vi "QueueToCommand.vi"(0 "ROS":T1={"topic port"=1236, "Node"="/labview", "topic"="/robot/head/command_head_nod", "type"="std_msgs/Bool", "node port"=7000, "error "={"status"=FALSE, "code"=0, "source"=""}, "Direction"=enum."Publisher", "Update (ms)"=1, "FIFO size"=1}, 2 "Check":enum16{"Cmd+Write", "FIFO", "CMD", "CMD /wait"}(ring)) -> (3 "ROS out":T1={"topic port"=1236, "Node"="/labview", "topic"="/robot/head/command_head_nod", "type"="std_msgs/Bool", "node port"=7000, "error "={"status"=FALSE, "code"=0, "source"=""}, "Direction"=enum."Publisher", "Update (ms)"=1, "FIFO size"=1}, 4 "Command":string, 5 "Queue log":string, 6 "data":string)   [LabVIEW 2014]
doc: "Executes a command from the queue"
uses:
  SubVIs/_ROSControl.ctl
  SubVIs/_ROSDirection.ctl
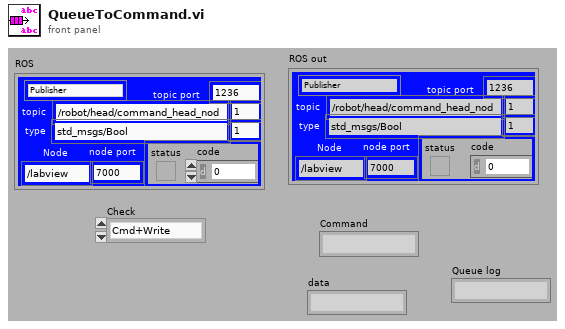
[diagram p1: front panel]
types:
  T1 = typedef "_ROSControl.ctl" = cluster{"topic port":u16, "Node":string, "topic":string, "type":string, "node port":u16, "error ":errorcluster, "Direction":T2, "Update (ms)":u16, "FIFO size":u16}
  T2 = typedef "_ROSDirection.ctl" = enum16{"Node", "Publisher", "Subscriber", "ServiceClient", "ServiceProvider"}
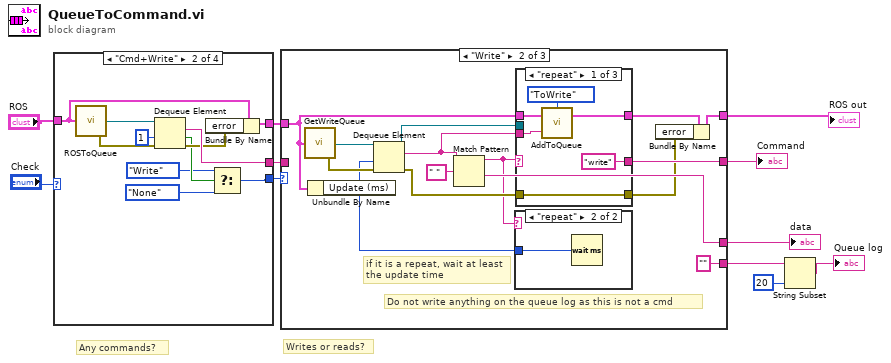
[diagram p0: block diagram]
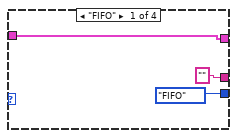
[diagram p2: hidden frame]
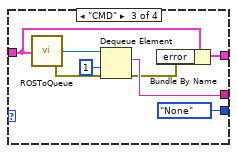
[diagram p3: hidden frame]
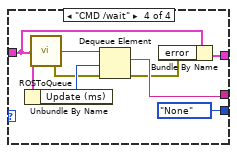
[diagram p4: hidden frame]
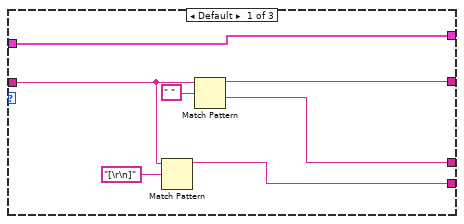
[diagram p5: hidden frame]
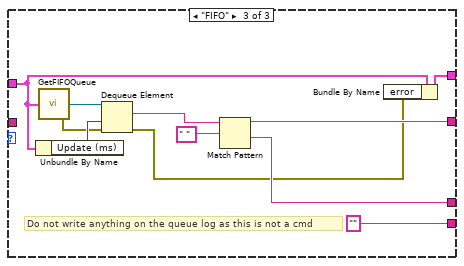
[diagram p9: hidden frame]
diagram:
  # "Writes or reads?"
  # "Any commands?"
  n1 = case shown="\"Cmd+Write\"" "Check" {
    tunnel: [enum16{"FIFO", "Write", "None"}."FIFO" w15 enum16{"FIFO", "Write", "None"}."None" enum16{"FIFO", "Write", "None"}."None"] -> w11
    tunnel: "ROS" -> [w13 w21 w29 w37]
    tunnel: ["" w23 w32 w40] -> w8
    tunnel: [w13 w20 w28 w36] -> w2
    frame "FIFO" {
    }
    frame "Cmd+Write" {
      n2 = call "ROSToQueue.vi"("ROS"=w21) -> ("error out"=w22:errorcluster, "queue"=w25:refnum<queue>)  [unwired: 3 in]
      n3 = Dequeue Element(queue=w25, timeout in ms (-1)=1, error in (no error)=w22) -> (element=w23:string, timed out?=w18:bool, error out=w19:errorcluster)  [unwired: 1 out]
      n4 = Bundle By Name(cluster=w21, "error"=w19) -> (w20:T1)
      n5 = Select(t=enum16{"FIFO", "Write", "None"}."Write", s=w18, f=enum16{"FIFO", "Write", "None"}."None") -> (s? t:f=w15:enum16{"FIFO", "Write", "None"})
    }
    frame "CMD" {
      n6 = call "ROSToQueue.vi"("ROS"=w29) -> ("error out"=w30:errorcluster, "queue"=w33:refnum<queue>)  [unwired: 3 in]
      n7 = Dequeue Element(queue=w33, timeout in ms (-1)=1, error in (no error)=w30) -> (element=w32:string, error out=w27:errorcluster)  [unwired: 2 out]
      n8 = Bundle By Name(cluster=w29, "error"=w27) -> (w28:T1)
    }
    frame "CMD /wait" {
      n9 = Unbundle By Name(w37) -> ("Update (ms)"=w39:u16)
      n10 = call "ROSToQueue.vi"("ROS"=w37) -> ("error out"=w38:errorcluster, "queue"=w41:refnum<queue>)  [unwired: 3 in]
      n11 = Dequeue Element(queue=w41, timeout in ms (-1)=w39, error in (no error)=w38) -> (element=w40:string, error out=w35:errorcluster)  [unwired: 2 out]
      n12 = Bundle By Name(cluster=w37, "error"=w35) -> (w36:T1)
    }
  }
  n13 = case shown="\"Write\"" w11 {
    tunnel: [w44 w62 w85] -> w10
    tunnel: [w43 "" ""] -> w6
    tunnel: [w45 w61 w84] -> w9
    tunnel: w8 -> [w46 _ _]
    tunnel: w2 -> [w42 w53 w81]
    tunnel: [w42 w57 w80] -> w1
    frame Default {
      n14 = Match Pattern(string=w46, regular expression="[\r\n]") -> (before substring=w43:string)  [unwired: 1 in, 3 out]
      n15 = Match Pattern(string=w46, regular expression=" ") -> (before substring=w45:string, after substring=w44:string)  [unwired: 1 in, 2 out]
    }
    frame "Write" {
      # "if it is a repeat, wait at least\nthe update time"
      # "Do not write anything on the queue log as this is not a cmd"
      n16 = call "GetWriteQueue.vi"("ROS"=w53) -> ("error out"=w51:errorcluster, "queue out"=w52:refnum<queue>)  [unwired: 3 in]
      n17 = Unbundle By Name(w53) -> ("Update (ms)"=w50:u16)
      n18 = Dequeue Element(queue=w52, timeout in ms (-1)=w50, error in (no error)=w51) -> (queue out=w56:refnum<queue>, element=w60:string, error out=w55:errorcluster)  [unwired: 1 out]
      n19 = Match Pattern(string=w60, regular expression=" ") -> (before substring=w49:string, after substring=w62:string)  [unwired: 1 in, 2 out]
      n20 = case shown="\"repeat\"" w49 {
        tunnel: w50 -> [_ w64]
        frame Default {
        }
        frame "repeat" {
          n21 = Wait (ms)(milliseconds to wait=w64) -> ()  [unwired: 1 out]
        }
      }
      n22 = case shown="\"repeat\"" w49 {
        selector: w49 -> [_ w73 w76]
        tunnel: ["write" w73 w76] -> w61
        tunnel: w53 -> [w69 w72 w75]
        tunnel: w60 -> [w68 _ _]
        tunnel: [w67 w72 w75] -> w58
        tunnel: w56 -> [_ _ _]
        tunnel: w55 -> [w66 w71 w74]
        tunnel: [w66 w71 w74] -> w54
        frame "repeat" {
          n23 = call "AddToQueue.vi"("Cmd"=w68, "ROS"=w69, "Type"=enum16{"topic", "node", "ToFIFO", "ToWrite"}."ToWrite") -> ("ROS out"=w67:T1)  [unwired: 2 in]
        }
        frame "write" {
        }
        frame Default {
        }
      }
      n24 = Bundle By Name(cluster=w58, "error"=w54) -> (w57:T1)
    }
    frame "FIFO" {
      # "Do not write anything on the queue log as this is not a cmd"
      n25 = Unbundle By Name(w81) -> ("Update (ms)"=w87:u16)
      n26 = call "GetFIFOQueue.vi"("ROS"=w81) -> ("error out"=w77:errorcluster, "queue out"=w78:refnum<queue>)  [unwired: 3 in]
      n27 = Dequeue Element(queue=w78, timeout in ms (-1)=w87, error in (no error)=w77) -> (element=w83:string, error out=w79:errorcluster)  [unwired: 2 out]
      n28 = Match Pattern(string=w83, regular expression=" ") -> (before substring=w84:string, after substring=w85:string)  [unwired: 1 in, 2 out]
      n29 = Bundle By Name(cluster=w81, "error"=w79) -> (w80:T1)
    }
  }
  "Command" <- w9
  "data" <- w10
  "ROS out" <- w1
  n30 = String Subset(string=w6, length (rest)=20 ("length (rest)")) -> (substring=→"Queue log":string)  [unwired: 1 in]
